vi "CreateTask.vi"(8 "error in":errorcluster, 11 "MainFGV_data":T1={"TestDir"=path "", "TestName"="", "task"="", "data_file"=refnum, "burts_file"=refnum, "log_file"=refnum, "AcqQueue"=refnum, "StartTime"=timestamp(0 s since 1904-01-01), "config_channels"=[], "DAQmx Device"="", "Advanced"={"rate"=1652.0, "duration"=1.0, "thr"=100.0, "preTrigger"=100.0, "cutoff"=-3.0, "Filtro"=enum."Desativado", "highPass"=1000.0, "lowPass"=1000.0, "updateTime"=50.0}, "running"=FALSE} {"Advanced"."updateTime" format="%#_g ms"; "Advanced"."lowPass" format="%#_g Hz"; "Advanced"."highPass" format="%#_g Hz"; "Advanced"."cutoff" format="%#_g dB"; "Advanced"."preTrigger" format="%#_g ms"; "Advanced"."thr" format="%#_g N"; "Advanced"."duration" format="%#_g s"; "Advanced"."rate" min=1652.0 max=51200.0 format="%#_g Hz"}) -> (0 "error out":errorcluster, 3 "MainFGV_data out":T1={"TestDir"=path "", "TestName"="", "task"="", "data_file"=refnum, "burts_file"=refnum, "log_file"=refnum, "AcqQueue"=refnum, "StartTime"=timestamp(0 s since 1904-01-01), "config_channels"=[], "DAQmx Device"="", "Advanced"={"rate"=1652.0, "duration"=1.0, "thr"=100.0, "preTrigger"=100.0, "cutoff"=-3.0, "Filtro"=enum."Desativado", "highPass"=1000.0, "lowPass"=1000.0, "updateTime"=50.0}, "running"=FALSE} {"Advanced"."updateTime" format="%#_g ms"; "Advanced"."lowPass" format="%#_g Hz"; "Advanced"."highPass" format="%#_g Hz"; "Advanced"."cutoff" format="%#_g dB"; "Advanced"."preTrigger" format="%#_g ms"; "Advanced"."thr" format="%#_g N"; "Advanced"."duration" format="%#_g s"; "Advanced"."rate" min=1652.0 max=51200.0 format="%#_g Hz"})   [LabVIEW 2016]
uses:
  MainFGV_data.ctl
  config_board.ctl
  Advanced/AdvancedConfig.ctl
  <vilib>/DAQmx/create/channels.llb/DAQmx Create Channel (AI-Acceleration-Accelerometer).vi
  <vilib>/DAQmx/create/channels.llb/DAQmx Create Channel (AI-Force-IEPE Sensor).vi
  <resource>/objmgr/daqmx.rc
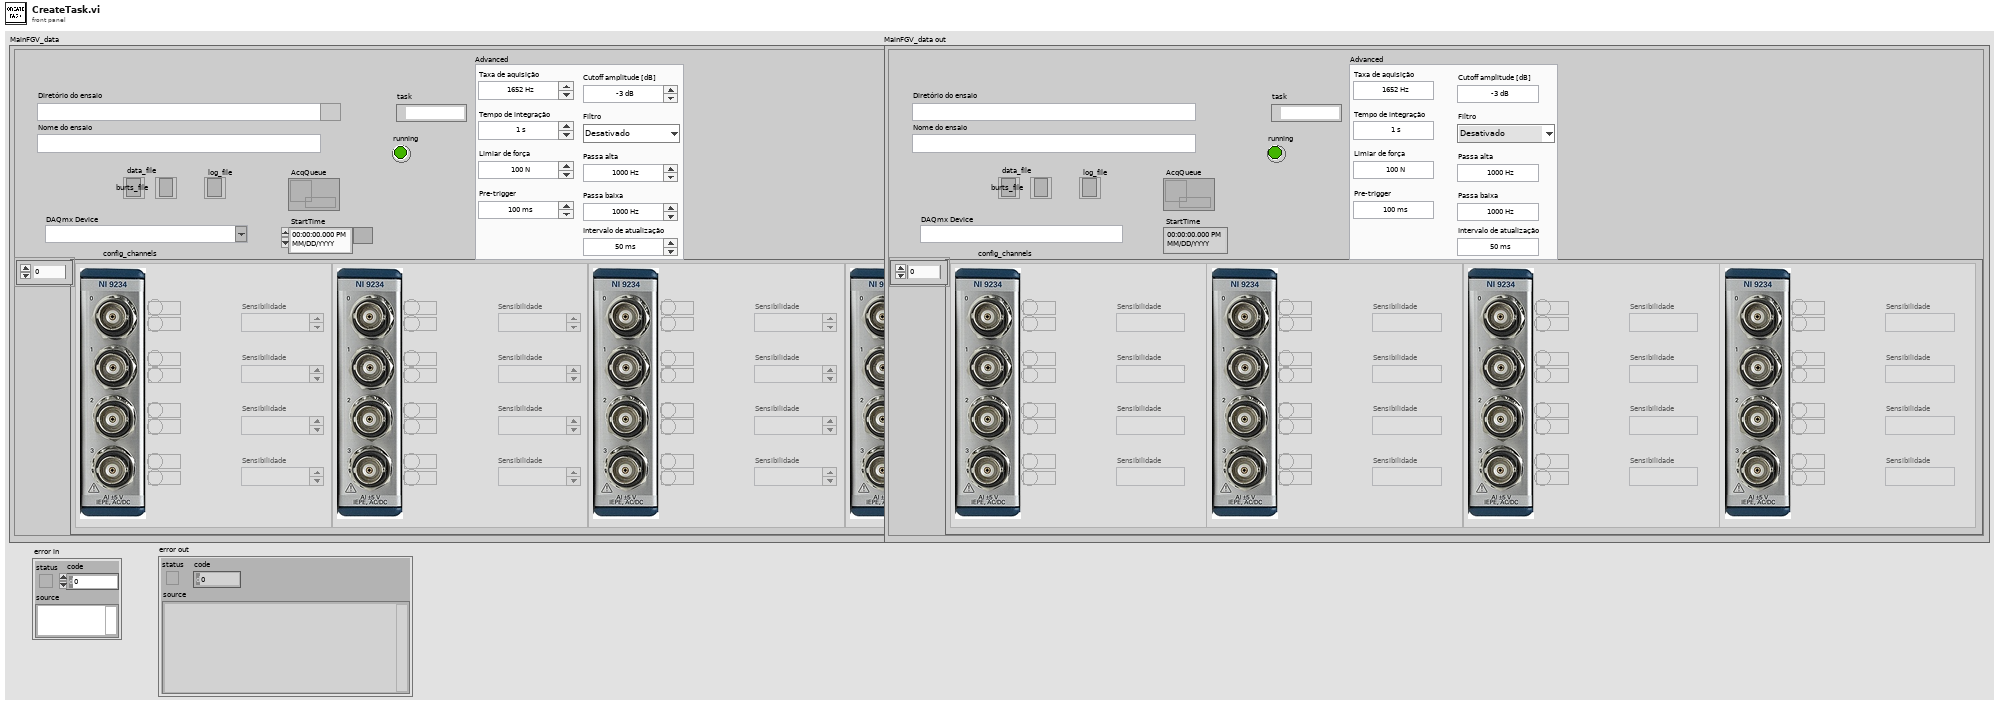
[diagram p1: front panel]
types:
  T1 = typedef "MainFGV_data.ctl" = cluster{"TestDir":path, "TestName":string, "task":refnum<k21>, "data_file":refnum<file>, "burts_file":refnum<file>, "log_file":refnum<file>, "AcqQueue":refnum<queue>, "StartTime":timestamp, "config_channels":T2[], "DAQmx Device":tag, "Advanced":T3, "running":bool}
  T2 = typedef "config_board.ctl" = cluster{"Sens 1":dbl, "active 1":bool, "type 1":bool, "type 2":bool, "active 2":bool, "Sens 2":dbl, "type 3":bool, "active 3":bool, "Sens 3":dbl, "type 4":bool, "active 4":bool, "Sens 4":dbl}
  T3 = typedef "AdvancedConfig.ctl" = cluster{"rate":dbl, "duration":dbl, "thr":dbl, "preTrigger":dbl, "cutoff":dbl, "Filtro":enum16{"Desativado", "Passa banda", "Passa alta", "Passa baixa"}, "highPass":dbl, "lowPass":dbl, "updateTime":dbl}
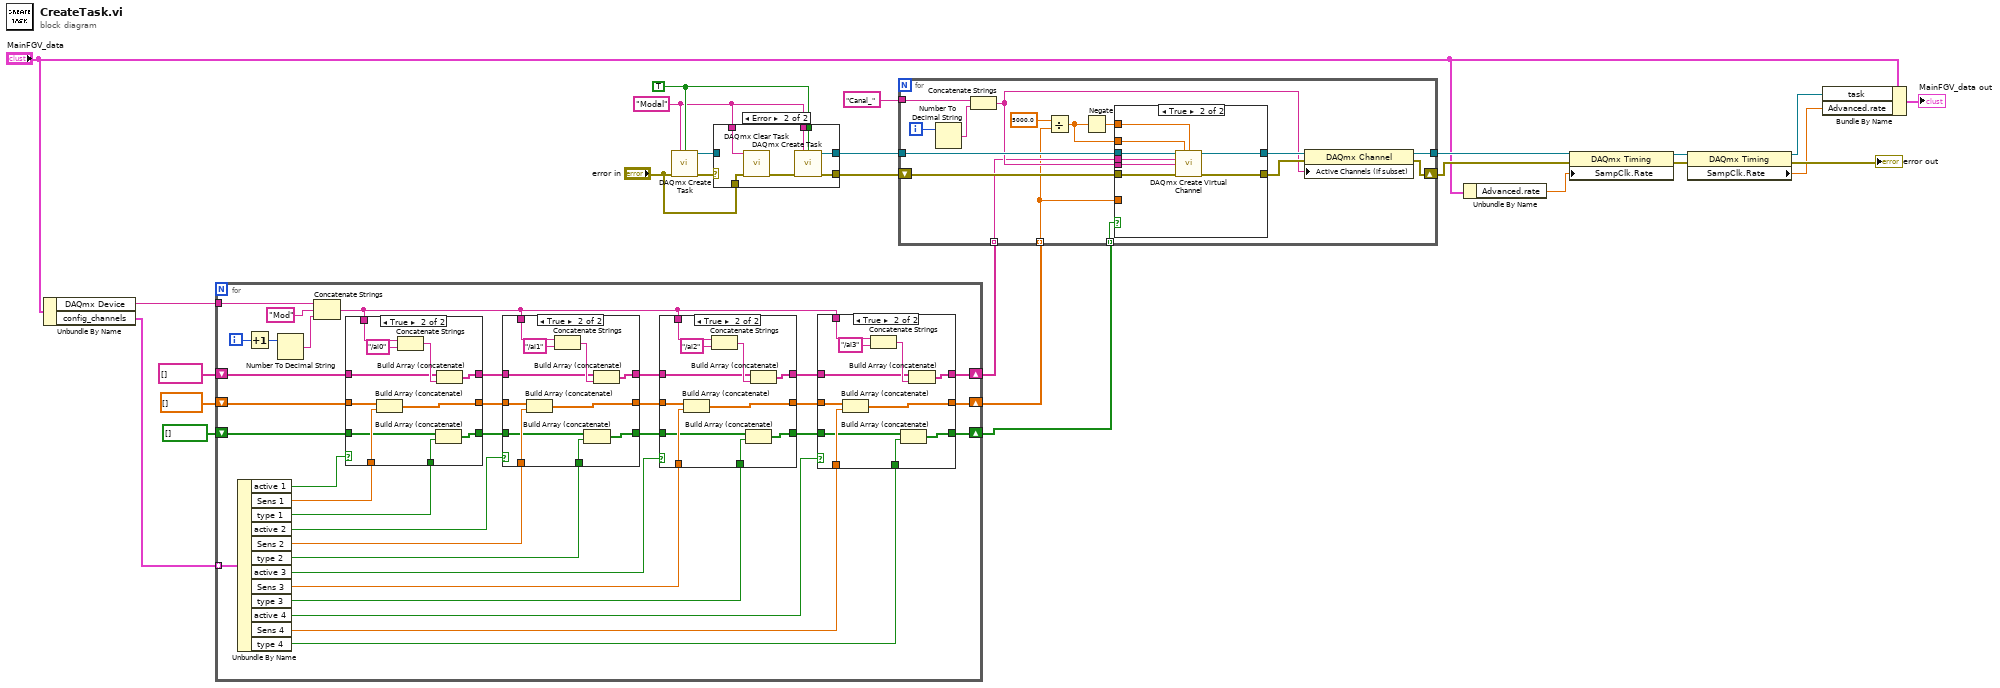
[diagram p0: block diagram]
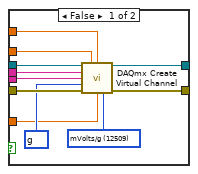
[diagram p6: hidden frame]
diagram:
  w22 = TRUE ("auto cleanup")
  w21 = "Modal" ("new task name")
  n1 = Unbundle By Name("MainFGV_data") -> ("DAQmx Device"=w10:tag, "config_channels"=w11:T2[])
  n2 = for {
    tunnel: w11 -> [w44] mode=indexing
    tunnel: w10 -> [w59]
    shift-right: [w46] -> w15
    shift-left: string[] [] -> [w55]
    shift-right: [w45] -> w14
    shift-left: dbl[] [] ("Sensibilidades [mV/g]") -> [w54]
    shift-right: [w28] -> w1
    shift-left: bool[] [] -> [w27]
    i -> [w60]
    n3 = Unbundle By Name(w44) -> ("active 1"=w43:bool, "Sens 1"=w42:dbl, "type 1"=w36:bool, "active 2"=w41:bool, "Sens 2"=w40:dbl, "type 2"=w33:bool, "active 3"=w39:bool, "Sens 3"=w34:dbl, "type 3"=w31:bool, "active 4"=w37:bool, "Sens 4"=w38:dbl, "type 4"=w29:bool)
    n4 = Increment(x=w60) -> (x+1=w57:i32)
    n5 = Number To Decimal String(number=w57) -> (decimal integer string=w56:string)  [unwired: 1 in]
    n6 = Concatenate Strings(w59, "Mod" ("string"), w56) -> (w51:string)
    n7 = case shown="True" w43 {
      tunnel: w51 -> [_ w116]
      tunnel: w55 -> [w105 w113]
      tunnel: w54 -> [w104 w112]
      tunnel: w42 -> [_ w109]
      tunnel: [w105 w111] -> w53
      tunnel: [w104 w110] -> w47
      tunnel: w36 -> [_ w108]
      tunnel: [w103 w107] -> w35
      tunnel: w27 -> [w103 w106]
      frame False {
      }
      frame True {
        n8 = Build Array (concatenate)(w112, w109) -> (w110:dbl[])
        n9 = Concatenate Strings(w116, "/ai0" ("string")) -> (w114:string)
        n10 = Build Array (concatenate)(w106, w108) -> (w107:bool[])
        n11 = Build Array (concatenate)(w113, w114) -> (w111:string[])
      }
    }
    n12 = case shown="True" w41 {
      tunnel: w51 -> [_ w102]
      tunnel: w53 -> [w91 w99]
      tunnel: w47 -> [w90 w98]
      tunnel: w40 -> [_ w95]
      tunnel: [w91 w97] -> w52
      tunnel: [w90 w96] -> w48
      tunnel: w35 -> [w89 w94]
      tunnel: w33 -> [_ w93]
      tunnel: [w89 w92] -> w32
      frame False {
      }
      frame True {
        n13 = Build Array (concatenate)(w98, w95) -> (w96:dbl[])
        n14 = Concatenate Strings(w102, "/ai1" ("string")) -> (w100:string)
        n15 = Build Array (concatenate)(w94, w93) -> (w92:bool[])
        n16 = Build Array (concatenate)(w99, w100) -> (w97:string[])
      }
    }
    n17 = case shown="True" w39 {
      tunnel: w51 -> [_ w88]
      tunnel: w52 -> [w77 w85]
      tunnel: w48 -> [w76 w84]
      tunnel: w34 -> [_ w81]
      tunnel: [w77 w83] -> w50
      tunnel: [w76 w82] -> w49
      tunnel: w32 -> [w75 w80]
      tunnel: w31 -> [_ w79]
      tunnel: [w75 w78] -> w30
      frame False {
      }
      frame True {
        n18 = Build Array (concatenate)(w84, w81) -> (w82:dbl[])
        n19 = Concatenate Strings(w88, "/ai2" ("string")) -> (w86:string)
        n20 = Build Array (concatenate)(w80, w79) -> (w78:bool[])
        n21 = Build Array (concatenate)(w85, w86) -> (w83:string[])
      }
    }
    n22 = case shown="True" w37 {
      tunnel: w51 -> [_ w74]
      tunnel: w50 -> [w63 w71]
      tunnel: w49 -> [w62 w70]
      tunnel: w38 -> [_ w67]
      tunnel: [w63 w69] -> w46
      tunnel: [w62 w68] -> w45
      tunnel: w30 -> [w61 w66]
      tunnel: w29 -> [_ w65]
      tunnel: [w61 w64] -> w28
      frame False {
      }
      frame True {
        n23 = Build Array (concatenate)(w70, w67) -> (w68:dbl[])
        n24 = Concatenate Strings(w74, "/ai3" ("string")) -> (w72:string)
        n25 = Build Array (concatenate)(w66, w65) -> (w64:bool[])
        n26 = Build Array (concatenate)(w71, w72) -> (w69:string[])
      }
    }
  }
  n27 = call <vilib>:"DAQmx Create Task.vi"("new task name"=w21, "auto cleanup"=w22, "error in"="error in") -> ("task out"=w24:refnum<k21>, "error out"=w25:errorcluster)  [unwired: 11 in]
  n28 = case shown="Error" w25 {
    selector: w25 -> [w117 _]
    tunnel: w24 -> [w118 _]
    tunnel: [w118 w120] -> w8
    tunnel: "error in" -> [_ w125]
    tunnel: [w117 w123] -> w9
    tunnel: w22 -> [_ w122]
    tunnel: w21 -> [_ w121]
    tunnel: w21 -> [_ w119]
    frame No Error {
    }
    frame Error {
      n29 = call <vilib>:"DAQmx Clear Task.vi"("task in"=w119, "error in"=w125) -> ("error out"=w124:errorcluster)  [unwired: 13 in]
      n30 = call <vilib>:"DAQmx Create Task.vi"("new task name"=w121, "auto cleanup"=w122, "error in"=w124) -> ("task out"=w120:refnum<k21>, "error out"=w123:errorcluster)  [unwired: 11 in]
    }
  }
  n31 = for {
    tunnel: w8 -> [w141]
    shift-right: [w133] -> w20
    shift-left: w9 -> [w140]
    tunnel: [w135] -> w18
    tunnel: w14 -> [w130] mode=indexing
    tunnel: "Canal_" ("new task name") -> [w137]
    tunnel: w15 -> [w131] mode=indexing
    tunnel: w1 -> [w126] mode=indexing
    i -> [w139]
    n32 = Number To Decimal String(number=w139) -> (decimal integer string=w138:string)  [unwired: 1 in]
    n33 = Concatenate Strings(w137, w138) -> (w132:string)
    n34 = Divide(x=5000.0 ("y"), y=w130) -> (x/y=w128:dbl)
    n35 = Negate(x=w128) -> (-x=w127:dbl)
    n36 = case shown="True" w126 {
      tunnel: w141 -> [w152 w160]
      tunnel: w140 -> [w151 w156]
      tunnel: [w150 w159] -> w136
      tunnel: [w149 w155] -> w134
      tunnel: w132 -> [w148 w153]
      tunnel: w131 -> [w147 w154]
      tunnel: w130 -> [w144 _]
      tunnel: w128 -> [w143 w158]
      tunnel: w127 -> [w142 w157]
      frame False {
        w145 = 10186 items=["g"=10186, "m/s^2"=12470, "in/s^2"=12471, "From Custom Scale"=10065] ("units")
        w146 = 12509 items=["mVolts/g"=12509, "Volts/g"=12510] ("sensitivity units")
        n37 = call-poly <vilib>:"DAQmx Create Virtual Channel.vi"("task in"=w152, "maximum value"=w143, "minimum value"=w142, "physical channels"=w147, "name to assign"=w148, "units"=w145, "error in"=w151, "sensitivity"=w144, "sensitivity units"=w146) -> ("task out"=w150:refnum<k21>, "error out"=w149:errorcluster)  [unwired: 5 in]
      }
      frame True {
        n38 = call-poly <vilib>:"DAQmx Create Virtual Channel.vi"("task in"=w160, "maximum value"=w158, "minimum value"=w157, "physical channels"=w154, "name to assign"=w153, "error in"=w156) -> ("task out"=w159:refnum<k21>, "error out"=w155:errorcluster)  [unwired: 8 in]
      }
    }
    n39 = property class="DAQmx Channel"(reference=w136, error in=w134, "Active Channels (if subset)"=w132) -> (reference out=w135:refnum<k21>, error out=w133:errorcluster)
  }
  n40 = Unbundle By Name("MainFGV_data") -> ("Advanced.rate"=w3:dbl)
  n41 = property class="DAQmx Timing"(reference=w18, error in=w20, "SampClk.Rate"=w3) -> (reference out=w13:refnum<k21>, error out=w12:errorcluster)
  n42 = property class="DAQmx Timing"(reference=w13, error in=w12) -> (reference out=w6:refnum<k21>, error out=→"error out":errorcluster, "SampClk.Rate"=w5:dbl)
  n43 = Bundle By Name(cluster="MainFGV_data", "task"=w6, "Advanced.rate"=w5) -> (→"MainFGV_data out":T1)
